vi "Exemple_Metrics_Precision_Recall_Fscore_Support.vi"() -> ()   [LabVIEW 2020]
uses:
  Objet/3 - Model selection and evaluation/3.3 - Metrics and scoring/precision_rfs/Precision_RFS.vi
panel:
  out "Data":T1
  out "error out":errorcluster caption="sortie d'erreur"
  in  "precision_recall_fscore_support":T2={"beta"=1.0, "labels"=["pig", "dog", "cat"], "pos_label"={"dtype_pos_label"="int", "pos_label"="1"}, "average"="None", "warn_for"=["precision", "recall", "f-score"], "sample_weight"=[], "zero_division"={"dtype_zero_division"="str", "zero_division"="warn"}, "Returns"="precision"}
  in  "error in (no error)":errorcluster caption="entrée d'erreur (pas d'erreur)"
  in  "y_pred":string[][](array[string])=[["cat"], ["pig"], ["dog"], ["cat"], ["cat"], ["dog"]]
  in  "y_true":string[][](array[string])=[["cat"], ["dog"], ["pig"], ["cat"], ["dog"], ["pig"]]
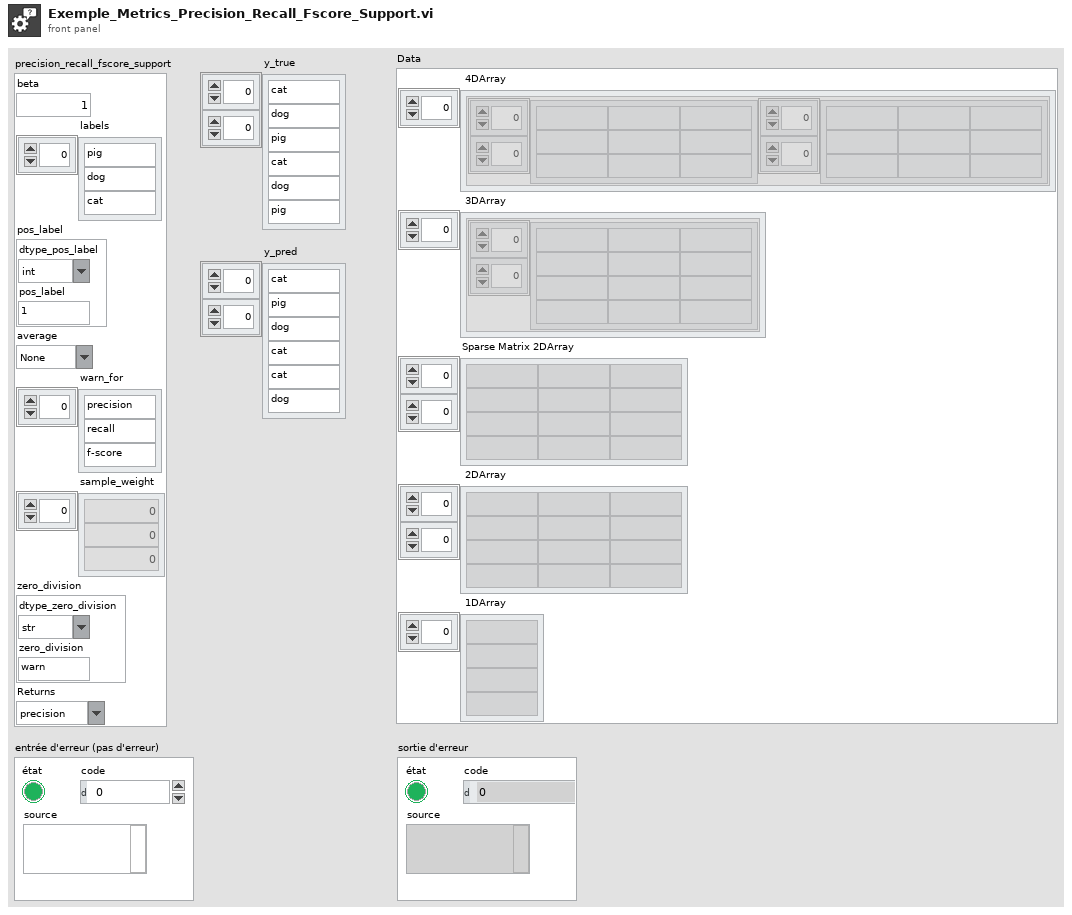
[diagram p1: front panel]
types:
  T1 = cluster{" 4DArray":cluster{"1":string[][], "2":string[][]}[], " 3DArray":cluster{"Tableau":string[][]}[], "Sparse Matrix 2DArray":string[][], " 2DArray":string[][], " 1DArray":string[]}
  T2 = cluster{"beta":dbl, "labels":string[], "pos_label":cluster{"dtype_pos_label":string, "pos_label":string}, "average":string, "warn_for":string[], "sample_weight":dbl[], "zero_division":cluster{"dtype_zero_division":string, "zero_division":string}, "Returns":string}
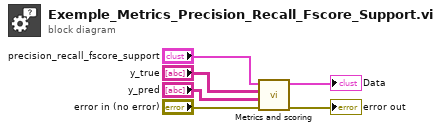
[diagram p0: block diagram]
diagram:
  n1 = call-poly "Metrics and scoring.vi"("error in (no error)"="error in (no error)", "y_pred"="y_pred", "y_true"="y_true", "precision_recall_fscore_support"="precision_recall_fscore_support") -> ("error out"=→"error out":errorcluster, "Data"=→"Data":T1)  [unwired: 6 in]
